vi "Example Loopback.vi"() -> ()   [LabVIEW 2013]
uses:
  C:/tf/play/labview/Tinkerforge.dll
  Tinkerforge.dll
panel:
  out "data":u8[](array[numeric])
  out "identifier":i64
  out "frameType":u8
  in  "stop":bool
  in  "uid":string="5556"
  in  "port":i32=4223
  in  "host":string="localhost"
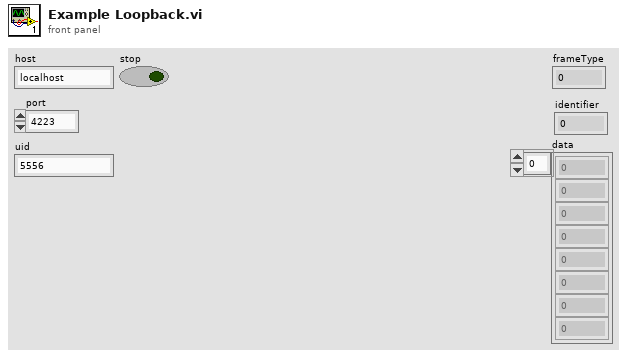
[diagram p1: front panel]
types:
  T1 = cluster{"data":u8[], "frameType":u8, "identifier":i64}
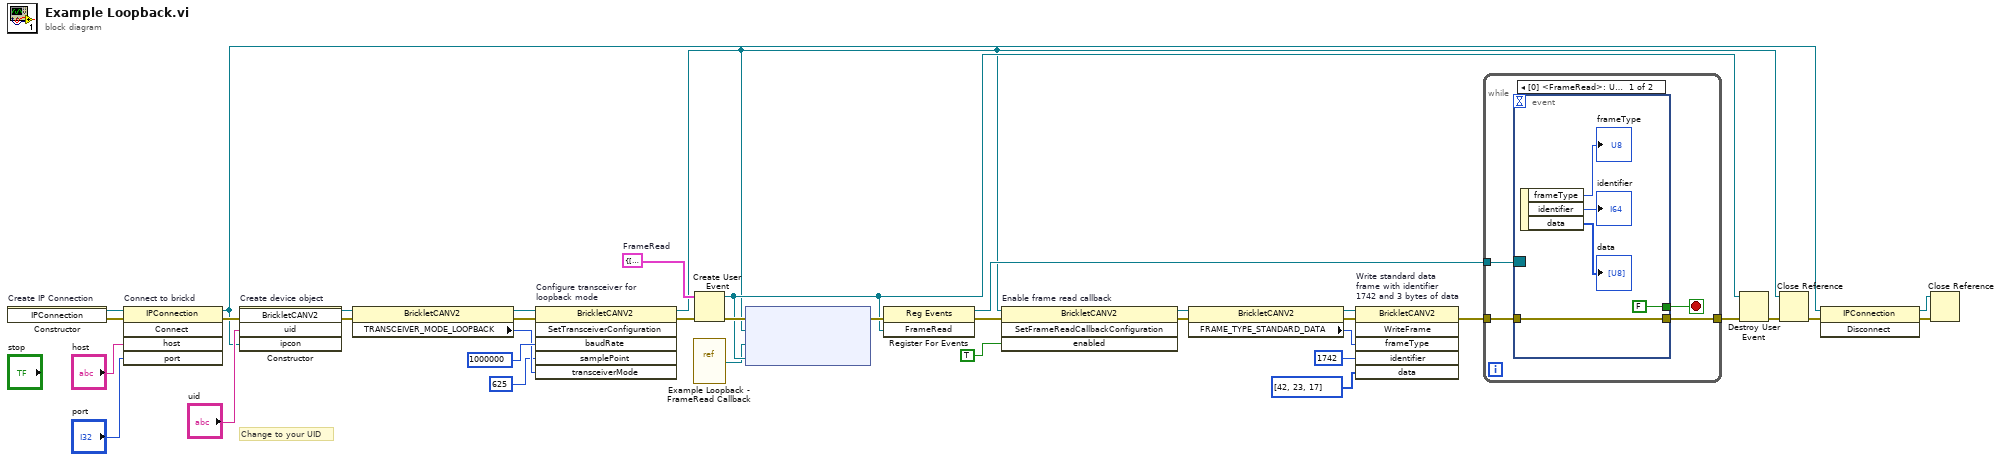
[diagram p0: block diagram]
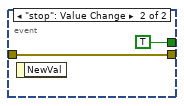
[diagram p2: hidden frame]
diagram:
  w21 = T1 {"data"=[], "frameType"=0, "identifier"=0}  # FrameRead
  # "Change to your UID"
  n1 = constructor on="Create IP Connection" class="IPConnection"() -> (reference out=w37:refnum<k24>, error out=w22:errorcluster)  [unwired: 3 in, 1 out]
  n2 = invoke on="Connect to brickd" class="IPConnection" method="Connect"(reference=w37, error in=w22, "host"="host", "port"="port") -> (reference out=w30:refnum<k24>, error out=w33:errorcluster)  [unwired: 1 in, 3 out]
  n3 = constructor on="Create device object" class="BrickletCANV2"(error in=w33, "uid"="uid", "ipcon"=w30) -> (reference out=w11:refnum<k24>, error out=w12:errorcluster)  [unwired: 2 in, 3 out]
  n4 = property class="BrickletCANV2"(reference=w11, error in=w12) -> (reference out=w7:refnum<k24>, error out=w8:errorcluster, "TRANSCEIVER_MODE_LOOPBACK"=w2:u8)
  n5 = invoke on="Configure transceiver for\nloopback mode" class="BrickletCANV2" method="SetTransceiverConfiguration"(reference=w7, error in=w8, "baudRate"=i64 1000000, "samplePoint"=625, "transceiverMode"=w2) -> (reference out=w10:refnum<k24>, error out=w9:errorcluster)  [unwired: 1 in, 4 out]
  n6 = vi-ref "Example Loopback - FrameRead Callback.vi"() -> ("vi reference"=w5:refnum<vi>)
  n7 = Create User Event(user event datatype=w21, error in=w9) -> (user event=w24:refnum<user-event>, error out=w28:errorcluster)
  n8 = node ("Register Event Callback")(w28, w10, w5, w24) -> (w27:errorcluster)  [unwired: 1 in, 1 out]
  n9 = register-events(error in=w27, w24) -> (reference out=w26:refnum<event-registration>, error out=w20:errorcluster)  [unwired: 1 in]
  n10 = invoke on="Enable frame read callback" class="BrickletCANV2" method="SetFrameReadCallbackConfiguration"(reference=w10, error in=w20, "enabled"=TRUE) -> (reference out=w18:refnum<k24>, error out=w16:errorcluster)  [unwired: 1 in, 2 out]
  n11 = property class="BrickletCANV2"(reference=w18, error in=w16) -> (reference out=w17:refnum<k24>, error out=w15:errorcluster, "FRAME_TYPE_STANDARD_DATA"=w14:u8)
  n12 = invoke on="Write standard data\nframe with identifier\n1742 and 3 bytes of data" class="BrickletCANV2" method="WriteFrame"(reference=w17, error in=w15, "frameType"=w14, "identifier"=i64 1742, "data"=u8[] [42, 23, 17]) -> (error out=w19:errorcluster)  [unwired: 1 in, 5 out]
  n13 = while {
    tunnel: w26 -> [w41]
    tunnel: [w40] -> w25
    tunnel: w19 -> [w39]
    stop <- w38 stop-if-true
    n14 = event shown="[0] <FrameRead>: User Event" {
      selector: w41 -> [_ _]
      dyn-events: _ -> [_ _]
      timeout: _ -> [_ _]
      tunnel: [w46 w47] -> w40
      tunnel: w39 -> [w46 w47]
      tunnel: [FALSE TRUE] -> w38
      event User Event {
        n15 = event-data() -> ("frameType"=→"frameType":u8, "identifier"=→"identifier":i64, "data"=→"data":u8[])  [unwired: 1 in]
      }
      event "stop": Value Change {
        n16 = event-data() -> ()  [unwired: 1 in, 1 out]
      }
    }
  }
  n17 = Destroy User Event(user event=w24, error in=w25) -> (error out=w23:errorcluster)
  n18 = Close Reference(reference=w10, error in (no error)=w23) -> (error out=w32:errorcluster)
  n19 = invoke class="IPConnection" method="Disconnect"(reference=w30, error in=w32) -> (reference out=w29:refnum<k24>, error out=w31:errorcluster)  [unwired: 1 in, 1 out]
  n20 = Close Reference(reference=w29, error in (no error)=w31) -> ()  [unwired: 1 out]
